vi "StageController.vi"() -> ()   [LabVIEW 2013]
panel:
  in  "moveForward":bool caption="Move Forward"
  in  "moveBackwards":bool caption="Move Backwards"
  in  "positions":string(combo) caption="Positions"
  in  "motorSpeed":dbl caption="Motor Speed (steps/s)" min=0.0 max=2000.0 format="%#.4g"
  in  "setEncodertoZero":bool caption="Set Encoder to Zero"
  in  "home":bool caption="Home"
  in  "motorCOM":refnum<visa-resource-name>="COM4" caption="Motor COM Port"
  in  "encoderCOM":refnum<visa-resource-name>="COM1" caption="Encoder COM Port"
  in  "showTerminal":bool caption="Show Terminal"
  in  "EXIT":bool
  out "currentPos":dbl caption="Current Position (mm)" format="%.3g"
  in  "goToSelPos":bool caption="Go to Selected Position"
  in  "selPos":dbl=1.0 caption="Selected Position  (mm)" min=1.0 max=4060.0 format="%.3g"
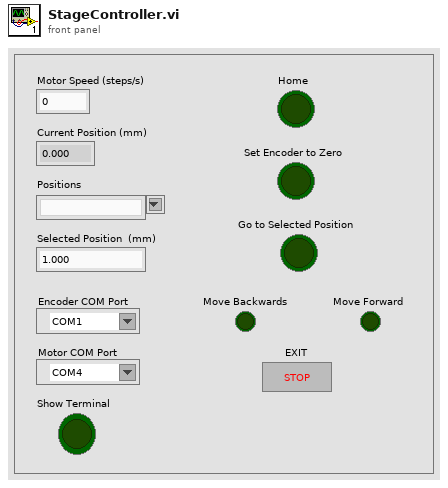
[diagram p1: front panel]
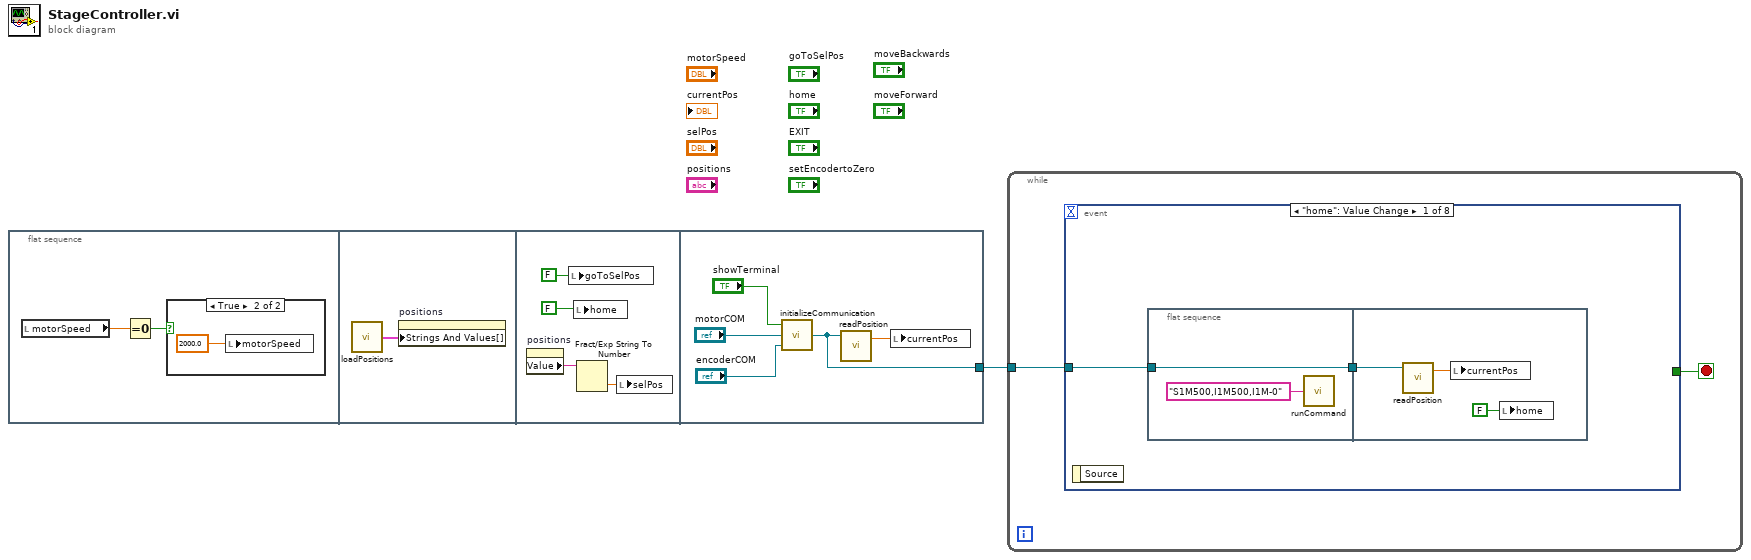
[diagram p0: block diagram]
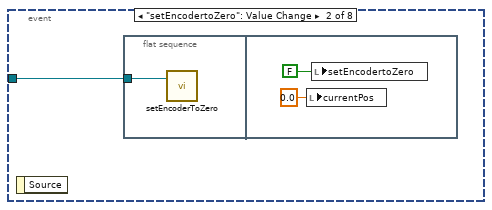
[diagram p3: hidden frame]
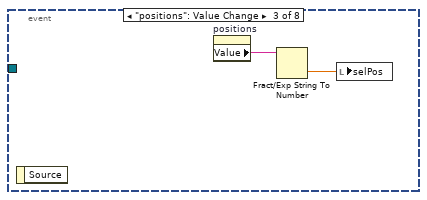
[diagram p4: hidden frame]
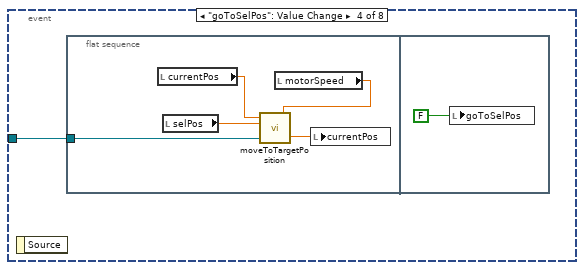
[diagram p5: hidden frame]
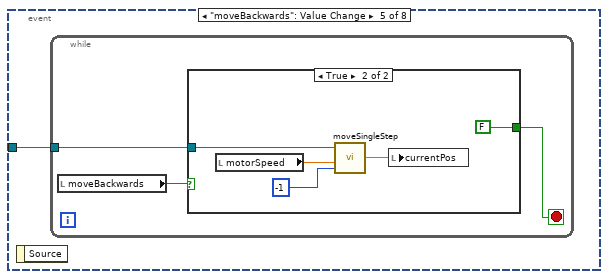
[diagram p6: hidden frame]
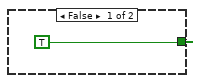
[diagram p7: hidden frame]
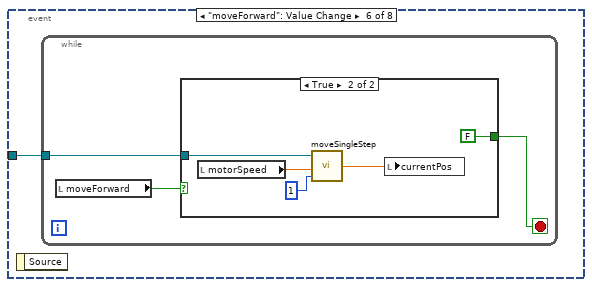
[diagram p8: hidden frame]
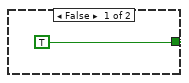
[diagram p9: hidden frame]
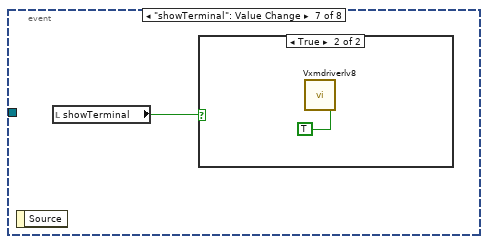
[diagram p10: hidden frame]
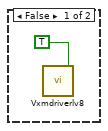
[diagram p11: hidden frame]
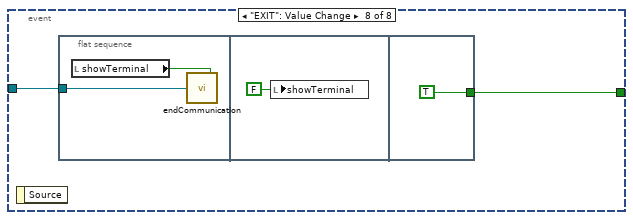
[diagram p12: hidden frame]
diagram:
  n1 = flat-sequence {
    tunnel: [w10] -> w1
    frame #0 {
      n2 = local read "motorSpeed"() -> (w2:dbl)
      n3 = Equal To 0?(x=w2) -> (x = 0?=w3:bool)
      n4 = case shown="True" w3 {
        frame False {
        }
        frame True {
          n5 = local write "motorSpeed"(2000.0 ("Motor Speed")) -> ()
        }
      }
    }
    frame #1 {
      n6 = call "loadPositions.vi"() -> ("positions"=w5:cluster{string, string}[])
      n7 = property on="positions" class="CmbBox"("Strings And Values[]"=w5) -> ()  [unwired: 2 in, 2 out]
    }
    frame #2 {
      n8 = property on="positions" class="CmbBox"() -> ("Value"=w7:string)  [unwired: 2 in, 2 out]
      n9 = local write "goToSelPos"(FALSE ("goToPos1")) -> ()
      n10 = local write "home"(FALSE ("Home")) -> ()
      n11 = Fract/Exp String To Number(string=w7) -> (number=w6:dbl)  [unwired: 3 in, 1 out]
      n12 = local write "selPos"(w6) -> ()
    }
    frame #3 {
      n13 = call "initializeCommunication.vi"("Encoder COM Port"="encoderCOM", "Motor COM Port"="motorCOM", "Show Terminal"="showTerminal") -> ("Encoder VISA Resource Name (out)"=w10:refnum<visa-resource-name>)
      n14 = call "readPosition.vi"("VISA resource name"=w10) -> ("position"=w11:dbl)  [unwired: 1 in, 2 out]
      n15 = local write "currentPos"(w11) -> ()
    }
  }
  n16 = while {
    tunnel: w1 -> [w16]
    stop <- w15 stop-if-true
    n17 = event shown="[0] \"home\": Value Change" {
      selector: _ -> [_ _ _ _ _ _ _ _]
      dyn-events: _ -> [_ _ _ _ _ _ _ _]
      timeout: _ -> [_ _ _ _ _ _ _ _]
      tunnel: w16 -> [w17 w24 _ w30 w37 w47 _ w61]
      tunnel: [_ _ _ _ _ _ _ w60] -> w15
      event "home": Value Change {
        n18 = event-data() -> ()  [unwired: 1 in, 1 out]
        n19 = flat-sequence {
          tunnel: [w19] -> w18
          tunnel: w17 -> [w19]
          tunnel: w18 -> [w21]
          frame #0 {
            n20 = call "runCommand.vi"("command"="S1M500,I1M500,I1M-0") -> ()  [unwired: 1 in]
          }
          frame #1 {
            n21 = call "readPosition.vi"("VISA resource name"=w21) -> ("position"=w22:dbl)  [unwired: 1 in, 2 out]
            n22 = local write "currentPos"(w22) -> ()
            n23 = local write "home"(FALSE ("Home")) -> ()
          }
        }
      }
      event "setEncodertoZero": Value Change {
        n24 = event-data() -> ()  [unwired: 1 in, 1 out]
        n25 = flat-sequence {
          tunnel: w24 -> [w25]
          frame #0 {
            n26 = call "setEncoderToZero.vi"("VISA resource name"=w25) -> ()  [unwired: 1 in, 2 out]
          }
          frame #1 {
            n27 = local write "currentPos"(0.0 ("currentPos")) -> ()
            n28 = local write "setEncodertoZero"(FALSE ("Set Encoder to Zero")) -> ()
          }
        }
      }
      event "positions": Value Change {
        n29 = event-data() -> ()  [unwired: 1 in, 1 out]
        n30 = property on="positions" class="CmbBox"() -> ("Value"=w29:string)  [unwired: 2 in, 2 out]
        n31 = Fract/Exp String To Number(string=w29) -> (number=w28:dbl)  [unwired: 3 in, 1 out]
        n32 = local write "selPos"(w28) -> ()
      }
      event "goToSelPos": Value Change {
        n33 = event-data() -> ()  [unwired: 1 in, 1 out]
        n34 = flat-sequence {
          tunnel: w30 -> [w32]
          frame #0 {
            n35 = local read "currentPos"() -> (w35:dbl)
            n36 = local read "selPos"() -> (w31:dbl)
            n37 = local read "motorSpeed"() -> (w33:dbl)
            n38 = call "moveToTargetPosition.vi"("speed"=w33, "Encoder COM Port"=w32, "targetPos"=w31, "currentPos"=w35) -> ("updatedCurrentPos"=w34:dbl)
            n39 = local write "currentPos"(w34) -> ()
          }
          frame #1 {
            n40 = local write "goToSelPos"(FALSE ("goToPos3")) -> ()
          }
        }
      }
      event "moveBackwards": Value Change {
        n41 = event-data() -> ()  [unwired: 1 in, 1 out]
        n42 = while {
          tunnel: w37 -> [w39]
          stop <- w40 stop-if-true
          n43 = local read "moveBackwards"() -> (w38:bool)
          n44 = case shown="True" w38 {
            tunnel: [TRUE FALSE] -> w40
            tunnel: w39 -> [_ w45]
            frame False {
            }
            frame True {
              n45 = local read "motorSpeed"() -> (w42:dbl)
              n46 = call "moveSingleStep.vi"("direction"=-1, "motorSpeed"=w42, "VISA resource name"=w45) -> ("position"=w43:dbl)
              n47 = local write "currentPos"(w43) -> ()
            }
          }
        }
      }
      event "moveForward": Value Change {
        n48 = event-data() -> ()  [unwired: 1 in, 1 out]
        n49 = while {
          tunnel: w47 -> [w48]
          stop <- w50 stop-if-true
          n50 = local read "moveForward"() -> (w49:bool)
          n51 = case shown="True" w49 {
            tunnel: [TRUE FALSE] -> w50
            tunnel: w48 -> [_ w55]
            frame False {
            }
            frame True {
              n52 = local read "motorSpeed"() -> (w52:dbl)
              n53 = call "moveSingleStep.vi"("direction"=1, "motorSpeed"=w52, "VISA resource name"=w55) -> ("position"=w53:dbl)
              n54 = local write "currentPos"(w53) -> ()
            }
          }
        }
      }
      event "showTerminal": Value Change {
        n55 = event-data() -> ()  [unwired: 1 in, 1 out]
        n56 = local read "showTerminal"() -> (w57:bool)
        n57 = case shown="True" w57 {
          frame False {
            n58 = call "Vxmdriverlv8.Vi"("Hide Terminal"=TRUE) -> ()  [unwired: 21 in, 6 out]
          }
          frame True {
            n59 = call "Vxmdriverlv8.Vi"("Show Terminal"=TRUE) -> ()  [unwired: 21 in, 6 out]
          }
        }
      }
      event "EXIT": Value Change {
        n60 = event-data() -> ()  [unwired: 1 in, 1 out]
        n61 = flat-sequence {
          tunnel: w61 -> [w63]
          tunnel: [TRUE] -> w60
          frame #0 {
            n62 = local read "showTerminal"() -> (w62:bool)
            n63 = call "endCommunication.vi"("Show Terminal"=w62, "Encoder COM Port"=w63) -> ()
          }
          frame #1 {
            n64 = local write "showTerminal"(FALSE ("Show Terminal")) -> ()
          }
          frame #2 {
          }
        }
      }
    }
  }
